vi "Set (DBL).vi"(6 "ISOBUS address":T4=-1 caption="ISOBUS address (-1)", 7 "Unit":T1, 8 "error in":errorcluster, 9 "Command Value (Dbl)":dbl format="%#.4g", 10 "SCPI Message(s)":string[](array[string]), 11 "Mercury Reference In":T5) -> (0 "error out":errorcluster, 2 "Response":T2, 3 "Mercury Reference Out":T5, 4 "Valid?":T3)   [LabVIEW 2019, in "Mercury iXX.lvlib"]
doc: "Write the selected value as a Dbl to the specified command on the remote instrument."
uses:
  Mercury iXX.lvlib
  Public/Controls/Mercury Reference.ctl
  Public/Controls/Comms Transport Layer.ctl
  Controls/Query Dynamic Reference.ctl
  Public/Controls/ISOBus Address.ctl
  Public/Controls/Is Valid LED.ctl
  Public/Controls/Response String.ctl
  Public/Controls/Unit String.ctl
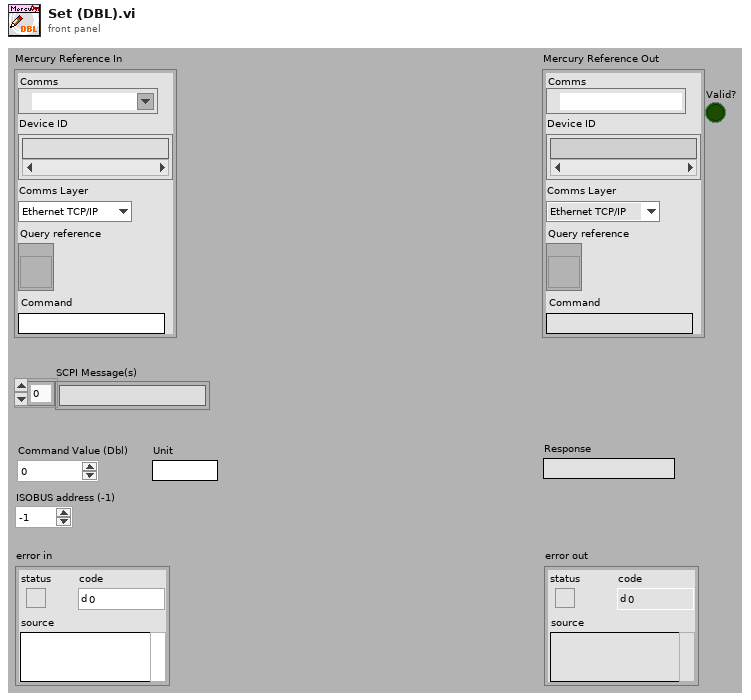
[diagram p1: front panel]
types:
  T1 = typedef "Mercury iXX.lvlib/Unit String.ctl" = string
  T2 = typedef "Mercury iXX.lvlib/Response String.ctl" = string
  T3 = typedef "Mercury iXX.lvlib/Is Valid LED.ctl" = bool
  T4 = typedef "Mercury iXX.lvlib/ISOBus Address.ctl" = i32
  T5 = typedef "Mercury iXX.lvlib/Mercury Reference.ctl" = cluster{"Comms":refnum<visa-resource-name>, "Device ID":string[], "Comms Layer":T6, "Command":string, "Query reference":T7}
  T6 = typedef "Mercury iXX.lvlib/Comms Transport Layer.ctl" = enum16{"Ethernet TCP/IP", "USB", "ISOBus - RS-232", "GPIB"}
  T7 = typedef "Mercury iXX.lvlib/Query Dynamic Reference.ctl" = refnum<vi>
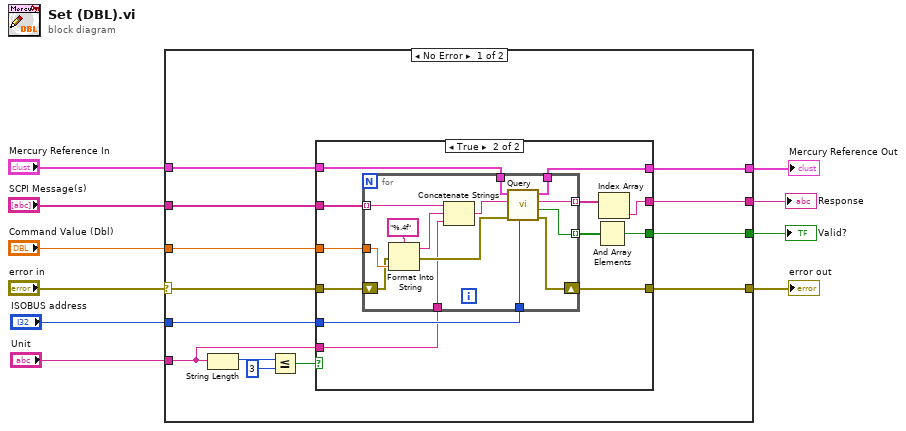
[diagram p0: block diagram]
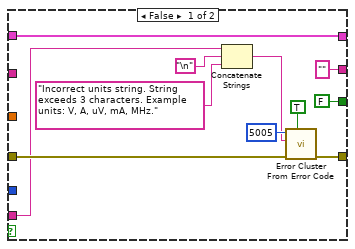
[diagram p2: hidden frame]
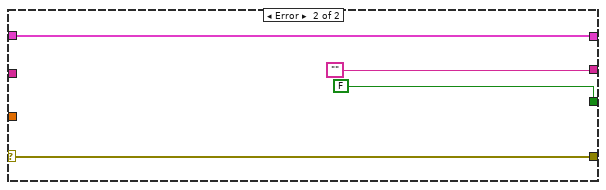
[diagram p3: hidden frame]
diagram:
  n1 = case shown="No Error" "error in" {
    selector: "error in" -> [w22 w63]
    tunnel: "Mercury Reference In" -> [w20 w64]
    tunnel: [w19 w64] -> w9
    tunnel: [w16 w63] -> w8
    tunnel: "ISOBUS address" -> [w21 _]
    tunnel: [w18 ""] -> w4
    tunnel: [w17 FALSE ("Valid?")] -> w5
    tunnel: "Command Value (Dbl)" -> [w23 _]
    tunnel: "SCPI Message(s)" -> [w15 _]
    tunnel: "Unit" -> [w11 _]
    frame No Error {
      n2 = String Length(string=w11) -> (length=w14:i32)
      n3 = Less Or Equal?(x=w14, y=3) -> (x <= y?=w12:bool)
      n4 = case shown="True" w12 {
        tunnel: w23 -> [_ w44]
        tunnel: w22 -> [w33 w43]
        tunnel: w21 -> [_ w42]
        tunnel: w20 -> [w34 w41]
        tunnel: [w34 w40] -> w19
        tunnel: ["" ("Data") w39] -> w18
        tunnel: [FALSE w38] -> w17
        tunnel: [w26 w37] -> w16
        tunnel: w15 -> [_ w36]
        tunnel: w11 -> [w28 w35]
        frame False {
          n5 = Concatenate Strings(w28, "\n", "Incorrect units string. String exceeds 3 characters. Example units: V, A, uV, mA, MHz." ("string")) -> (w27:string)
          n6 = call <vilib>:"Error Cluster From Error Code.vi"("show call chain? (False)"=TRUE, "error in (no error)"=w33, "error message (\"\")"=w27, "error code (0)"=5005) -> ("error out"=w26:errorcluster)  [unwired: 5 out]
        }
        frame True {
          n7 = for {
            tunnel: w36 -> [w60] mode=indexing
            tunnel: w44 -> [w58]
            tunnel: [w55] -> w46 mode=indexing
            tunnel: w41 -> [w54]
            tunnel: [w53] -> w40
            tunnel: [w52] -> w45 mode=indexing
            tunnel: w42 -> [w51]
            shift-right: [w48] -> w37
            shift-left: w43 -> [w50]
            tunnel: w35 -> [w47]
            n8 = Format Into String(format string="%.4f", error in=w50, w58) -> (resulting string=w57:string, error out=w49:errorcluster)  [unwired: 1 in]
            n9 = Concatenate Strings(w60, w57, w47) -> (w56:string)
            n10 = call "Query.vi"("ISOBUS address"=w51, "error in"=w49, "Command"=w56, "Mercury Reference In"=w54) -> ("error out"=w48:errorcluster, "Valid?"=w52:bool, "Data"=w55:string, "Mercury Reference Out"=w53:T5)  [unwired: 1 in, 3 out]
          }
          n11 = And Array Elements(Boolean array=w45) -> (logical AND=w38:bool)
          n12 = Index Array(array=w46) -> (element=w39:string)  [unwired: 1 in]
        }
      }
    }
    frame Error {
    }
  }
  "Mercury Reference Out" <- w9
  "error out" <- w8
  "Valid?" <- w5
  "Response" <- w4
